vi "fgv_XYStage_Position.vi"(0 "Coordinates I/P":cluster{"X":sgl, "Y":sgl, "Z":sgl}, 3 "error in (no error)":errorcluster, 4 "Status":enum16{"Write", "Read"}(ring)) -> (7 "Coordinates O/P":cluster{"X":sgl, "Y":sgl, "Z":sgl}, 10 "error out":errorcluster)   [LabVIEW 2020]
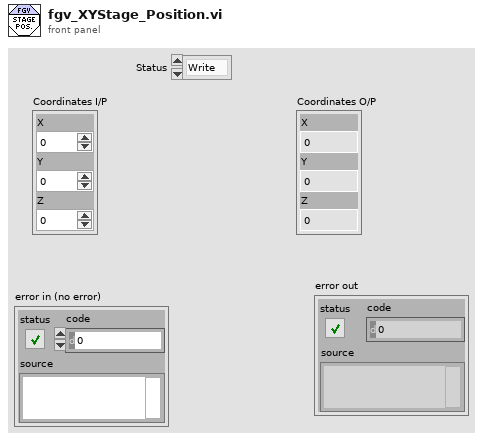
[diagram p1: front panel]
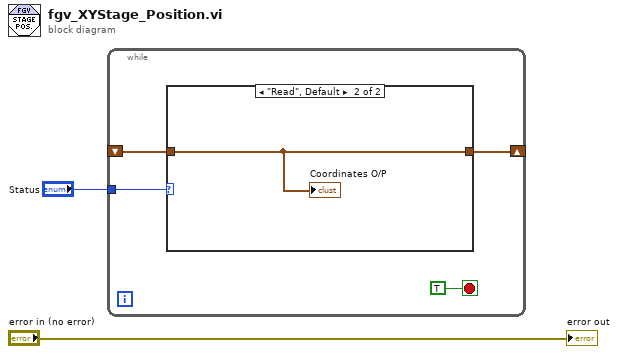
[diagram p0: block diagram]
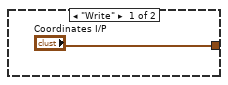
[diagram p2: hidden frame]
diagram:
  n1 = while {
    tunnel: "Status" -> [w5]
    shift-right: [w4] -> _
    shift-left: _ -> [w3]
    stop <- TRUE stop-if-true
    n2 = case shown="\"Read\", Default" w5 {
      tunnel: ["Coordinates I/P" w8] -> w4
      tunnel: w3 -> [_ w8]
      frame "Write" {
      }
      frame "Read", Default {
        "Coordinates O/P" <- w8
      }
    }
  }
  "error out" <- "error in (no error)"
